vi "SequenceIndexWrite.vi"(8 "error in (no error)":errorcluster, 9 "OriginalName":string, 10 "SequenceIndex":refnum<class "SequenceIndex.lvclass">, 11 "VariableManagerRef in":refnum<vi>) -> (0 "error out":errorcluster, 3 "VariableManagerRef out":refnum<vi>)   [LabVIEW 2013, in "VariableManagerAPI.lvlib"]
doc: "Add the given sequence index definition to database.\nTo overwrite existing sequence index definition, provide the OriginalName.\n\nAn error is thrown if the given SequenceIndex is malformed, failing the test in SequenceIndexCheck.vi\n\nSuppose that a sequence index has a name <B>idx</B>. Three names are reserved for uses in sequence function\n<B>idx</B>: Integer value that runs from 0 to (idx.Steps-1)\n<B>idx_f</B>: Double value that runs [0,1] (gives 0, if the idx.Steps is 1)\n<B>idx_max</B>: An integer equals to idx.Steps"
uses:
  VariableManagerAPI.lvlib
  VariableManager/VariableManager.lvclass
  SequenceIndex/SequenceIndex.lvclass
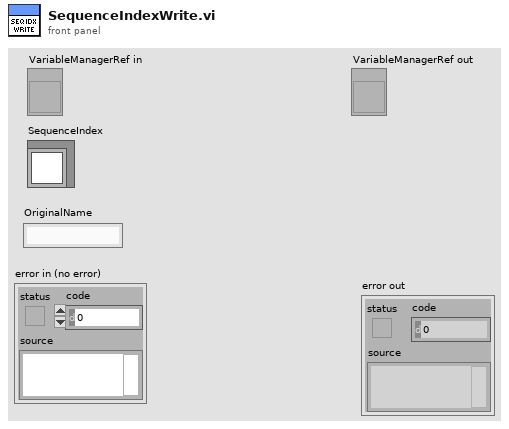
[diagram p1: front panel]
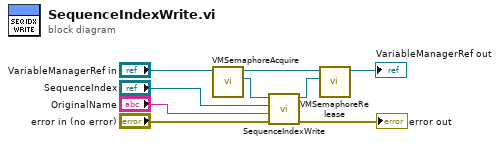
[diagram p0: block diagram]
diagram:
  n1 = call "VMSemaphoreAcquire.vi"("VariableManagerRef in"="VariableManagerRef in") -> ("VariableManager"=w6:refnum<class "VariableManager.lvclass">, "VariableManagerRef out"=w8:refnum<vi>)  [unwired: 7 in, 2 out]
  n2 = call-dynamic "SequenceIndexWrite.vi"("error in (no error)"="error in (no error)", "OriginalName"="OriginalName", "SequenceIndex"="SequenceIndex", "VariableManager in"=w6) -> ("error out"=→"error out":errorcluster, "VariableManager out"=w5:refnum<class "VariableManager.lvclass">)  [unwired: 6 in]
  n3 = call "VMSemaphoreRelease.vi"("VariableManager"=w5, "VariableManagerRef in"=w8) -> ("VariableManagerRef out"=→"VariableManagerRef out":refnum<vi>)  [unwired: 8 in, 1 out]
